vi "FTW-Router-Worker.vi"(1 "Endpoint":refnum<class "FTW-Endpoint.lvclass">, 2 "Message Handler":refnum<user-event>) -> ()   [LabVIEW 2013, in "FTW-Router.lvclass"]
uses:
  FTW-Router.lvclass
  Message/Request/FTW-Message-IncomingRequest.lvclass
  Endpoint/FTW-Endpoint.lvclass
panel:
  out "Messages Handled":u32
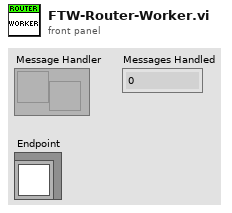
[diagram p1: front panel]
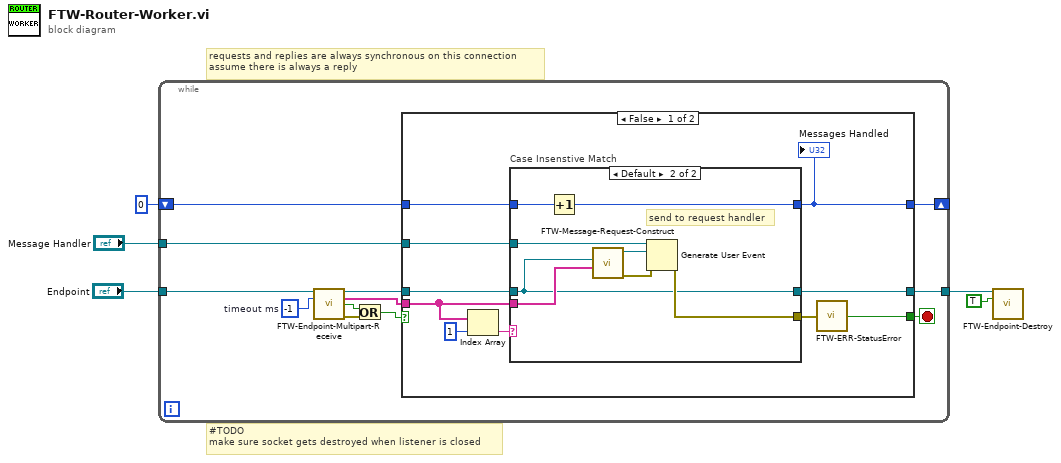
[diagram p0: block diagram]
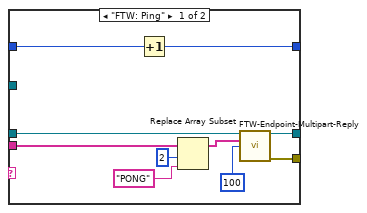
[diagram p2: hidden frame]
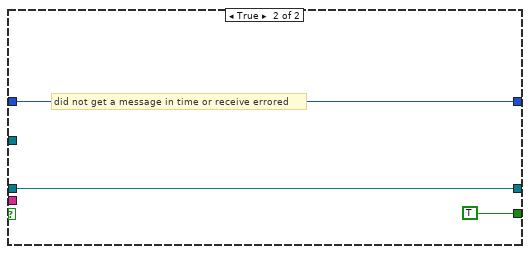
[diagram p3: hidden frame]
diagram:
  # "#TODO\nmake sure socket gets destroyed when listener is closed"
  # "requests and replies are always synchronous on this connection\nassume there is always a reply"
  n1 = while {
    tunnel: "Message Handler" -> [w17]
    shift-right: [w10] -> _
    shift-left: u32 0 -> [w11]
    tunnel: "Endpoint" -> [w16]
    tunnel: [w6] -> w3
    stop <- w12 stop-if-true
    w15 = -1  # timeout ms
    n2 = call-dynamic "FTW-Endpoint-Multipart-Receive.vi"("FTW Endpoint"=w16, "Timeout"=w15) -> ("FTW Endpoint out"=w9:refnum<class "FTW-Endpoint.lvclass">, "Message Received"=w13:string[], "Timed out?"=w7:bool, "error out"=w14:errorcluster)  [unwired: 10 in]
    n3 = Or(x=w7, y=w14) -> (x .or. y?=w8:bool)
    n4 = case shown="False" w8 {
      tunnel: w17 -> [w27 _]
      tunnel: w13 -> [w23 _]
      tunnel: [w20 TRUE] -> w12
      tunnel: w9 -> [w24 w46]
      tunnel: w11 -> [w26 w48]
      tunnel: [w18 w48] -> w10
      tunnel: [w19 w46] -> w6
      frame False {
        n5 = Index Array(array=w23, index=1) -> (element=w21:string)
        n6 = case "Case Insenstive Match" shown="Default" w21 {
          tunnel: w27 -> [_ w45]
          tunnel: w26 -> [w37 w44]
          tunnel: [w28 w43] -> w18
          tunnel: [w36 w40] -> w25
          tunnel: w24 -> [w35 w38]
          tunnel: w23 -> [w33 w39]
          tunnel: [w34 w38] -> w19
          frame "FTW: Ping" {
            n7 = Increment(x=w37) -> (x+1=w28:u32)
            n8 = Replace Array Subset(array=w33, new element="PONG" ("Part"), index=2) -> (w32:string[])
            n9 = call-dynamic "FTW-Endpoint-Multipart-Reply.vi"("FTW Endpoint"=w35, "Multipart Message"=w32, "Timeout"=100) -> ("FTW Endpoint out"=w34:refnum<class "FTW-Endpoint.lvclass">, "error out"=w36:errorcluster)  [unwired: 10 in, 1 out]
          }
          frame Default {
            # "send to request handler"
            n10 = Increment(x=w44) -> (x+1=w43:u32)
            n11 = call "FTW-Message-Request-Construct.vi"("Multipart Message"=w39, "Frontend Endpoint"=w38) -> ("error out"=w42:errorcluster, "FTW Incoming Request"=w41:refnum<class "FTW-Message-IncomingRequest.lvclass">)  [unwired: 8 in]
            n12 = Generate User Event(user event=w45, event data cluster=w41, error in=w42) -> (error out=w40:errorcluster)  [unwired: 1 in, 1 out]
          }
        }
        "Messages Handled" <- w18
        n13 = call "FTW-ERR-StatusError.vi"("error to check"=w25) -> ("Error?"=w20:bool)
      }
      frame True {
        # "did not get a message in time or receive errored"
      }
    }
  }
  n14 = call-dynamic "FTW-Endpoint-Destroy.vi"("FTW Endpoint"=w3, "Force Destroy"=TRUE) -> ()  [unwired: 13 in, 1 out]
